vi "Practica_8.vi"() -> ()   [LabVIEW 2016]
panel:
  in  "Enum 3":enum16{""}(ring)
  in  "Enum 2":enum16{"Seno", "Coseno", ""}(ring)
  in  "Enum":enum16{"Seno", "Coseno", "Tangente"}(ring)
  in  "Muestras":i32(slide) scale=2.0..1000.0
  in  "Offet":dbl(knob) scale=-10.0..10.0
  in  "Fase":dbl(knob) scale=0.0..360.0
  in  "Frecuencia":dbl(knob) scale=0.0..15.0
  in  "Amplitud":dbl(knob) scale=-10.0..10.0
  out "Waveform Graph":dbl[](graph)
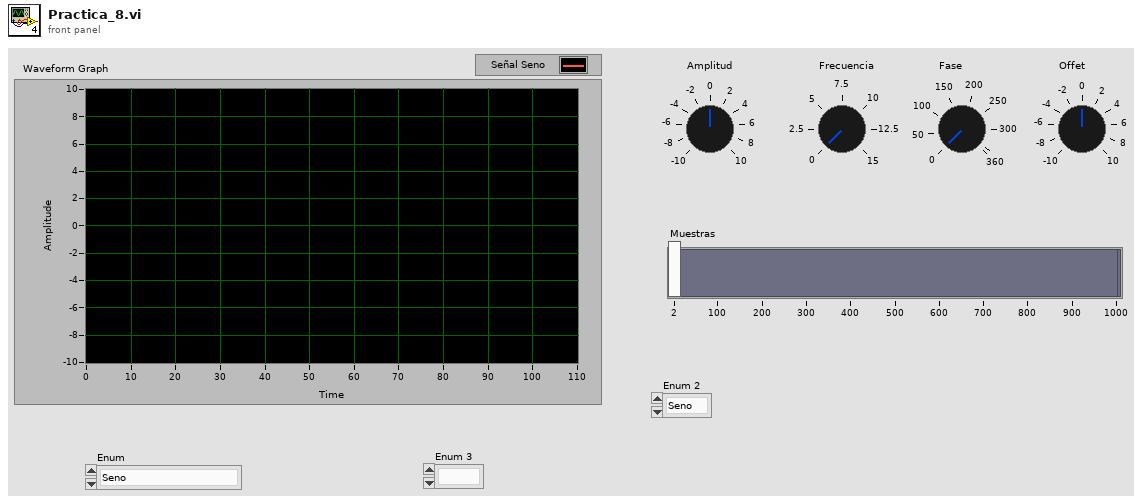
[diagram p1: front panel]
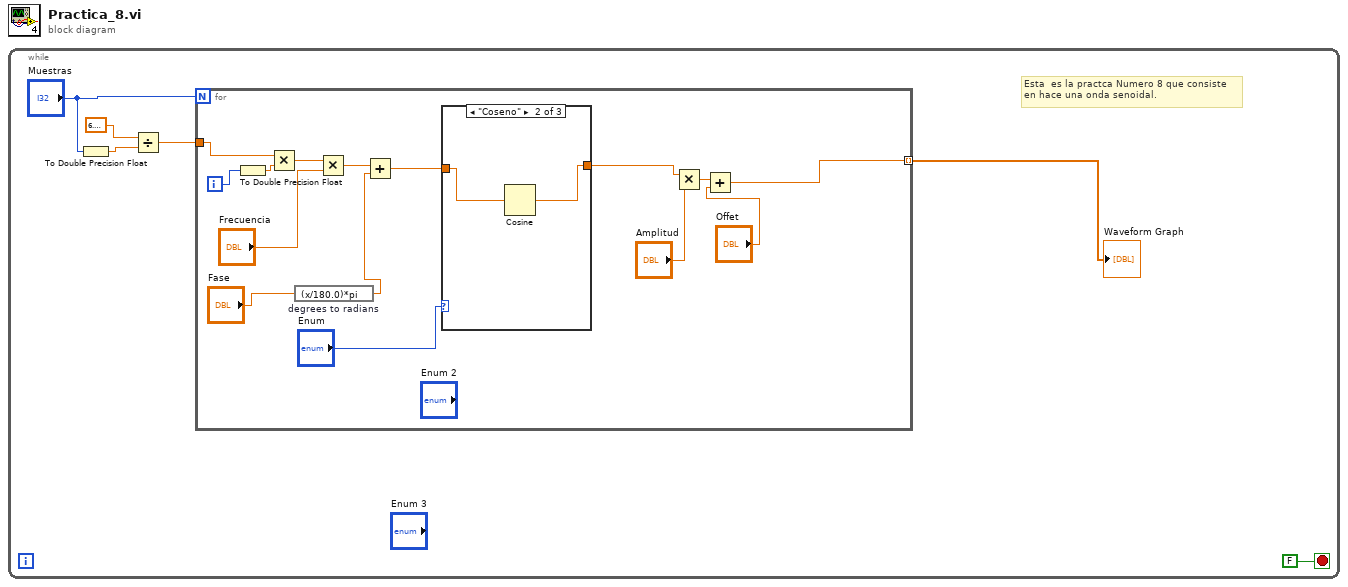
[diagram p0: block diagram]
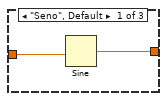
[diagram p2: hidden frame]
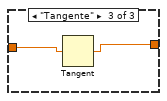
[diagram p3: hidden frame]
diagram:
  n1 = while {
    stop <- FALSE stop-if-true
    # "Esta  es la practca Numero 8 que consiste\nen hace una onda senoidal."
    n2 = To Double Precision Float(number="Muestras") -> (double precision float=w3:dbl)
    n3 = Divide(x=6.283185307179586, y=w3) -> (x/y=w2:dbl)
    n4 = for {
      N: "Muestras" -> [_]
      tunnel: w2 -> [w21]
      tunnel: [w17] -> w1 mode=indexing
      i -> [w19]
      n5 = To Double Precision Float(number=w19) -> (double precision float=w20:dbl)
      n6 = Multiply(x=w21, y=w20) -> (x*y=w12:dbl)
      n7 = expression code="(x/180.0)*pi" "degrees to radians"("Fase") -> (w8:dbl)
      n8 = Multiply(x=w12, y="Frecuencia") -> (x*y=w11:dbl)
      n9 = Add(x=w11, y=w8) -> (x+y=w10:dbl)
      n10 = case shown="\"Coseno\"" "Enum" {
        tunnel: [w23 w24 w27] -> w16
        tunnel: w10 -> [w22 w25 w26]
        frame "Seno", Default {
          n11 = Sine(x=w22) -> (sin(x)=w23:dbl)
        }
        frame "Coseno" {
          n12 = Cosine(x=w25) -> (cos(x)=w24:dbl)
        }
        frame "Tangente" {
          n13 = Tangent(1:w26) -> (0:w27:dbl)
        }
      }
      n14 = Multiply(x=w16, y="Amplitud") -> (x*y=w15:dbl)
      n15 = Add(x=w15, y="Offet") -> (x+y=w17:dbl)
    }
    "Waveform Graph" <- w1
  }
